vi "HaltTactic_v2_Init.vi"(0 "object in":refnum<class "HaltTactic_v2.lvclass">, 5 "error in (no error)":errorcluster) -> (14 "object out":refnum<class "HaltTactic_v2.lvclass">, 19 "error out":errorcluster)   [LabVIEW 2023, in "HaltTactic_v2.lvclass"]
uses:
  HaltTactic_v2.lvclass
  C:/Users/ebert/Documents/codes/SSL/repo/SSL_AI/NewSTP/NewTactics/Tactic_v2_class/Tactic_v2.lvclass
  NewSkills/HaltSkill_v2_class/HaltSkill_v2.lvclass
  C:/Users/ebert/Documents/codes/SSL/repo/SSL_AI/NewSTP/NewSkills/Skill_v2_class/Skill_v2.lvclass
  Tactic_v2_class/Tactic_v2.lvclass
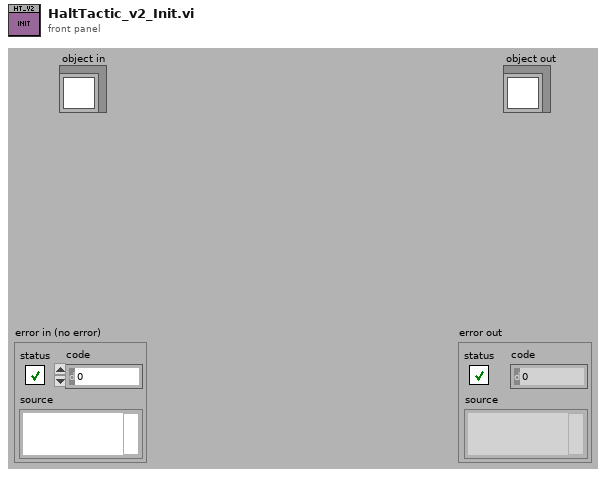
[diagram p1: front panel]
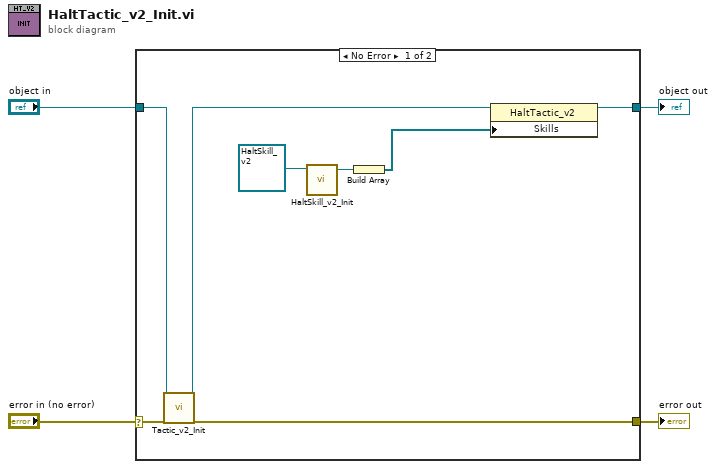
[diagram p0: block diagram]
diagram:
  n1 = case shown="No Error" "error in (no error)" {
    selector: "error in (no error)" -> [w12 w13]
    tunnel: [w8 w14] -> w4
    tunnel: "object in" -> [w10 w14]
    tunnel: [w11 w13] -> w1
    frame No Error {
      n2 = call "Tactic_v2_Init.vi"("object in"=w10, "error in (no error)"=w12) -> ("object out"=w9:refnum<class "HaltTactic_v2.lvclass">, "error out"=w11:errorcluster)  [unwired: 16 in]
      n3 = call "HaltSkill_v2_Init.vi"("object in"=refnum<class "HaltSkill_v2.lvclass"> refnum ("HaltSkill_v2")) -> ("object out"=w6:refnum<class "HaltSkill_v2.lvclass">)  [unwired: 17 in, 1 out]
      n4 = Build Array(w6) -> (w5:refnum<class "HaltSkill_v2.lvclass">[])
      n5 = property class="HaltTactic_v2"(reference=w9, "Skills"=w5) -> (reference out=w8:refnum<class "HaltTactic_v2.lvclass">)  [unwired: 1 in, 1 out]
    }
    frame Error {
    }
  }
  "object out" <- w4
  "error out" <- w1
